vi "Stream Status.vi"(8 "error in (no error)":errorcluster, 11 "OBS in":refnum<class "OBS.lvclass">) -> (0 "error out":errorcluster, 2 "Stream Status":T1, 3 "OBS out":refnum<class "OBS.lvclass">)   [LabVIEW 2022 SP3, in "obs-websocket-lv.lvlib" / "OBS.lvclass"]
uses:
  OBS.lvclass
  OBS.lvclass/OBS.ctl
  GetStreamStatus/GetStreamStatus.lvclass
  RGetStreamStatus/RGetStreamStatus.lvclass
  C:/dev/illuminatedg/obs-websocket-lv/obs-websocket-lv/Response/Response.lvclass
  C:/dev/illuminatedg/obs-websocket-lv/obs-websocket-lv/Server Message/Server Message.lvclass
  C:/dev/illuminatedg/obs-websocket-lv/obs-websocket-lv/Message/Message.lvclass
  C:/dev/illuminatedg/obs-websocket-lv/obs-websocket-lv/RGetStreamStatus/RGetStreamStatus.lvclass
  C:/dev/illuminatedg/obs-websocket-lv/obs-websocket-lv/Request/Request.lvclass
  C:/dev/illuminatedg/obs-websocket-lv/obs-websocket-lv/Client Message/Client Message.lvclass
  C:/dev/illuminatedg/obs-websocket-lv/obs-websocket-lv/GetStreamStatus/GetStreamStatus.lvclass
  Stream Status.ctl
  obs-websocket-lv.lvlib
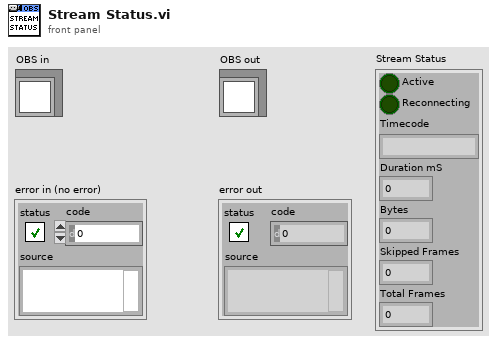
[diagram p1: front panel]
types:
  T1 = typedef "obs-websocket-lv.lvlib/Stream Status.ctl" = cluster{"Active":bool, "Reconnecting":bool, "Timecode":string, "Duration mS":u32, "Bytes":u32, "Skipped Frames":u32, "Total Frames":u32}
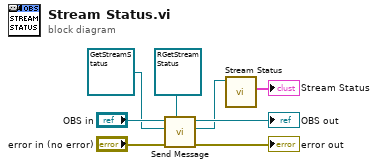
[diagram p0: block diagram]
diagram:
  n1 = call "Send Message.vi"("Response Type (None)"=refnum<class "RGetStreamStatus.lvclass"> refnum ("obs-websocket-lv.lvlib:RGetStreamStatus.lvclass"), "error in (no error)"="error in (no error)", "Client Message"=refnum<class "GetStreamStatus.lvclass"> refnum ("obs-websocket-lv.lvlib:GetStreamStatus.lvclass"), "OBS in"="OBS in") -> ("error out"=→"error out":errorcluster, "Response"=w2:refnum<class "RGetStreamStatus.lvclass">, "OBS out"=→"OBS out":refnum<class "OBS.lvclass">)  [unwired: 4 in, 1 out]
  n2 = call "Stream Status.vi"("RGetStreamStatus in"=w2) -> ("Stream Status"=→"Stream Status":T1)  [unwired: 8 in, 2 out]
